vi "GetAIDirection.vi"(8 "error in (no error)":errorcluster, 10 "SnakeGame in in":refnum<class "SnakeGame.lvclass">, 11 "AI_Snake in":refnum<class "AI_Snake.lvclass">) -> (0 "error out":errorcluster, 1 "Direction":T1, 2 "SnakeGame out":refnum<class "SnakeGame.lvclass">, 3 "AI_Snake out":refnum<class "AI_Snake.lvclass">)   [LabVIEW 2019, in "RT_Game.lvlib" / "AI_Snake.lvclass"]
uses:
  AI_Snake.lvclass
  SnakeGame/SnakeGame.lvclass
  C:/Users/FreshBob/Dropbox/VIs/myRIO_GameConsole/RT/RT_Game/Snake/Snake.lvclass
  Snake/Direction.ctl
  Snake/Snake.lvclass/Snake.ctl
  AI_Snake.lvclass/AI_Snake.ctl
  SnakeGame/SnakeGame.lvclass/SnakeGame.ctl
  SnakeGame/GridValue.ctl
  Snake/Read Position (Tiles).vi
  SnakeGame/Read Snakes.vi
  Snake/Read Length.vi
  SnakeGame/Read target_count.vi
  Snake/Snake.lvclass
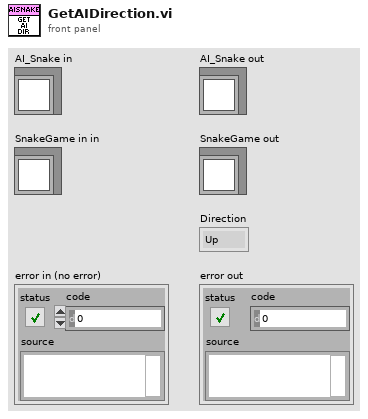
[diagram p1: front panel]
types:
  T1 = typedef "RT_Game.lvlib/Snake.lvclass/Direction.ctl" = enum16{"Up", "Left", "Down", "Right"}
  T2 = typedef "RT_Game.lvlib/Game.lvclass/Coordinate.ctl" = cluster{"x":dbl, "y":dbl}
  T3 = typedef "RT_Game.lvlib/Engine.lvclass/Coordinate.ctl" = cluster{"x":dbl, "y":dbl}
  T4 = typedef "RT_Game.lvlib/SnakeGame.lvclass/GridValue.ctl" = enum16{"Empty", "Snake1", "Snake1upLeft", "Snake1upRight", "Snake1downLeft", "Snake1downRight", "Snake2", "Snake2upLeft", "Snake2upRight", "Snake2downLeft", "Snake2downRight", "Score", "Speed", "Slow"}
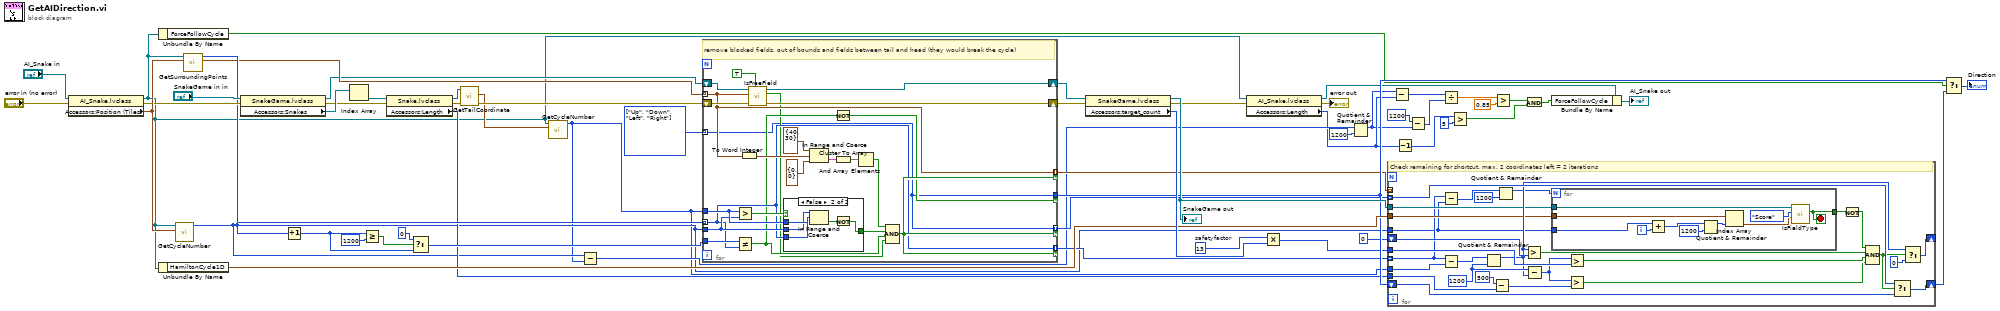
[diagram p0: block diagram]
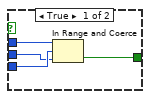
[diagram p2: hidden frame]
diagram:
  w36 = i16 13  # safetyfactor
  w41 = T1[] [enum."Up", enum."Down", enum."Left", enum."Right"] items=["Up", "Left", "Down", "Right"] ("Array")
  n1 = property class="AI_Snake.lvclass"(reference="AI_Snake in", error in="error in (no error)") -> (reference out=w16:refnum<class "AI_Snake.lvclass">, error out=w48:errorcluster, "Accessors:Position (Tiles)"=w51:T2)
  n2 = Unbundle By Name(w16) -> ("ForceFollowCycle"=w43:bool)
  n3 = Unbundle By Name(w16) -> ("HamiltonCycle1D"=w54:cluster{"x":i16, "y":i16}[])
  n4 = call "GetCycleNumber.vi"("coordinate"=w51, "AI_Snake in"=w16) -> ("CycleNumber"=w12:i16)  [unwired: 9 in]
  n5 = call "GetSurroundingPoints.vi"("Accessors:Position (Tiles)"=w51, "AI_Snake in"=w16) -> ("Array"=w39:T3[], "CycleValues"=w40:i16[])  [unwired: 8 in]
  n6 = property class="SnakeGame.lvclass"(reference="SnakeGame in in", error in=w48) -> (reference out=w35:refnum<class "SnakeGame.lvclass">, error out=w32:errorcluster, "Accessors:Snakes"=w33:refnum<class "Snake.lvclass">[])
  n7 = Increment(x=w12) -> (x+1=w28:i16)
  n8 = Index Array(array=w33) -> (element=w24:refnum<class "Snake.lvclass">)  [unwired: 1 in]
  n9 = Greater Or Equal?(x=w28, y=i16 1200) -> (x >= y?=w31:bool)
  n10 = property class="Snake.lvclass"(reference=w24, error in=w32) -> (reference out=w23:refnum<class "Snake.lvclass">, error out=w25:errorcluster, "Accessors:Length"=w22:i16)
  n11 = Select(t=i16 0, s=w31, f=w28) -> (s? t:f=w52:i16)
  n12 = call "GetTailCoordinate.vi"("error in (no error)"=w25, "Snake in"=w23) -> ("error out"=w50:errorcluster, "Coordinate"=w34:T3)  [unwired: 7 in, 1 out]
  n13 = call "GetCycleNumber.vi"("coordinate"=w34, "AI_Snake in"=w16) -> ("CycleNumber"=w11:i16)  [unwired: 9 in]
  n14 = Subtract(x=w12, y=w11) -> (x-y=w21:i16)
  n15 = for {
    tunnel: w39 -> [w76] mode=indexing
    shift-right: [w80] -> w56
    shift-left: w35 -> [w79]
    shift-right: [w78] -> w49
    shift-left: w50 -> [w77]
    tunnel: [w76] -> w45 mode=indexing if=w68
    tunnel: w40 -> [w64] mode=indexing
    tunnel: [w64] -> w44 mode=indexing if=w68
    tunnel: w41 -> [w59] mode=indexing
    tunnel: [w59] -> w46 mode=indexing if=w68
    tunnel: w12 -> [w69]
    tunnel: w11 -> [w70]
    tunnel: w52 -> [w65]
    tunnel: [w59] -> w53 if=w62
    # "remove blocked fields, out of bounds and fields between tail and head (they would break the cycle)"
    n16 = Greater?(x=w70, y=w69) -> (0:w66:bool)
    n17 = Not Equal?(x=w65, y=w64) -> (x != y?=w63:bool)
    n18 = To Word Integer(number=w76) -> (16bit integer=w75:cluster{"x":i16, "y":i16})
    n19 = call "IsFreeField.vi"("SnakesOnly?"=TRUE, "error in (no error)"=w77, "Coordinate"=w76, "SnakeGame in"=w79) -> ("error out"=w78:errorcluster, "Free?"=w60:bool, "SnakeGame out"=w80:refnum<class "SnakeGame.lvclass">)  [unwired: 5 in]
    n20 = case shown="False" w66 {
      tunnel: w64 -> [w85 w90]
      tunnel: w70 -> [w83 w89]
      tunnel: w69 -> [w82 w88]
      tunnel: [w84 w86] -> w67
      frame True {
        n21 = In Range and Coerce(upper limit=w83, x=w85, lower limit=w82) -> (In Range?=w84:bool)  [unwired: 1 out]
      }
      frame False {
        n22 = In Range and Coerce(upper limit=w88, x=w90, lower limit=w89) -> (In Range?=w87:bool)  [unwired: 1 out]
        n23 = Not(x=w87) -> (.not. x?=w86:bool)
      }
    }
    n24 = In Range and Coerce(upper limit=cluster{"x":i16, "y":i16} {"x"=40, "y"=30}, x=w75, lower limit=cluster{"x":i16, "y":i16} {"x"=0, "y"=0}) -> (In Range?=w61:cluster{"x":bool, "y":bool})  [unwired: 1 out]
    n25 = Not(x=w63) -> (.not. x?=w62:bool)
    n26 = Cluster To Array(cluster=w61) -> (array=w72:bool[])
    n27 = And Array Elements(Boolean array=w72) -> (logical AND=w71:bool)
    n28 = Compound Arithmetic op=AND(w71, w67, w63, w60) -> (w68:bool)
  }
  n29 = property class="SnakeGame.lvclass"(reference=w56, error in=w49) -> (reference out=w57:refnum<class "SnakeGame.lvclass">, error out=w55:errorcluster, "Accessors:target_count"=w58:i16)
  "SnakeGame out" <- w57
  n30 = property class="AI_Snake.lvclass"(reference=w16, error in=w55) -> (reference out=w15:refnum<class "AI_Snake.lvclass">, error out=→"error out":errorcluster, "Accessors:Length"=w8:i16)
  n31 = Multiply(x=w36, y=w58) -> (x*y=w20:i16)
  n32 = Quotient & Remainder(x=w21, y=i16 1200) -> (x-y*floor(x/y)=w5:i16)  [unwired: 1 out]
  n33 = for {
    tunnel: w45 -> [_] mode=indexing
    tunnel: w44 -> [w98] mode=indexing
    tunnel: w11 -> [w116]
    tunnel: w20 -> [w117]
    shift-right: [w113] -> w37
    shift-left: w53 -> [w114]
    tunnel: w46 -> [w111] mode=indexing
    shift-right: [w104] -> _
    shift-left: i16 0 ("t") -> [w110]
    tunnel: w54 -> [w107]
    tunnel: w12 -> [w97]
    tunnel: w57 -> [w106]
    tunnel: w22 -> [w91]
    w118 = i16 1200 ("y")
    # "Check remaining for shortcut. max. 2 coordinates left = 2 iterations"
    n34 = Subtract(x=w98, y=w97) -> (x-y=w100:i16)
    n35 = Subtract(x=w98, y=w116) -> (x-y=w115:i16)
    n36 = Quotient & Remainder(x=w115, y=w118) -> (x-y*floor(x/y)=w108:i16)  [unwired: 1 out]
    n37 = Subtract(x=i16 500 ("y"), y=w91) -> (x-y=w92:i16)
    n38 = Quotient & Remainder(x=w100, y=i16 1200) -> (x-y*floor(x/y)=w96:i16)  [unwired: 1 out]
    n39 = Greater?(x=w108, y=w110) -> (0:w109:bool)
    n40 = Subtract(x=w118, y=w108) -> (x-y=w94:i16)
    n41 = for {
      N: w96 -> [_]
      tunnel: w97 -> [w127]
      tunnel: w107 -> [w126]
      tunnel: w106 -> [w124]
      tunnel: [w121] -> w102
      i -> [w128]
      stop <- w121 stop-if-true
      n42 = Add(x=w127, y=w128) -> (x+y=w125:i32)
      n43 = Quotient & Remainder(x=w125, y=1200 ("x")) -> (x-y*floor(x/y)=w119:i32)  [unwired: 1 out]
      n44 = Index Array(array=w126, index=w119) -> (element=w122:cluster{"x":i16, "y":i16})
      n45 = call "IsFieldType.vi"("Coordinate"=w122, "Type"=GridValue."Score", "SnakeGame in"=w124) -> ("IsType?"=w121:bool)  [unwired: 6 in, 2 out]
    }
    n46 = Greater?(x=w94, y=w117) -> (0:w112:bool)
    n47 = Greater?(x=w94, y=w92) -> (0:w95:bool)
    n48 = Not(x=w102) -> (.not. x?=w105:bool)
    n49 = Compound Arithmetic op=AND(w105, w109, w112, w95) -> (w101:bool)
    n50 = Select(t=w111, s=w101, f=w114) -> (s? t:f=w113:T1)
    n51 = Select(t=w108, s=w101, f=i16 0 ("t")) -> (s? t:f=w104:i16)
  }
  n52 = Subtract(x=w5, y=w8) -> (x-y=w3:i16)
  n53 = Decrement(x=w8) -> (x-1=w9:i16)
  n54 = Subtract(x=i16 1200 ("y"), y=w5) -> (x-y=w4:i16)
  n55 = Divide(x=w3, y=w4) -> (x/y=w2:dbl)
  n56 = Greater?(x=w9, y=i16 5) -> (0:w13:bool)
  n57 = Greater?(x=w2, y=0.85) -> (0:w7:bool)
  n58 = And(x=w7, y=w13) -> (x .and. y?=w14:bool)
  n59 = Bundle By Name(cluster=w15, "ForceFollowCycle"=w14) -> (→"AI_Snake out":refnum<class "AI_Snake.lvclass">)
  n60 = Select(t=w53, s=w43, f=w37) -> (s? t:f=→"Direction":T1)
